vi "Audio Playback.vi"() -> ()   [LabVIEW 2020]
uses:
  support/typedefs/Playback_States.ctl
  support/typedefs/Audio CFG.ctl
  <vilib>/Dataflow_G/G-Audio/Controls/Audio File Info.ctl
  <vilib>/sound2/lvsound2.llb/Sound Output Task ID.ctl
  <vilib>/sound2/lvsound2.llb/Sampling Mode.ctl
  <vilib>/sound2/lvsound2.llb/Sound Data Format.ctl
  <vilib>/Dataflow_G/G-Audio/G-Audio.lvlib
panel:
  in  "Stop":bool
  out "#Samples":u64 format="#Samples: %d"
  in  "Audio Timeline":dbl(slide)=1.0 max=100.0 scale=0.0..100.0 scale format="%#_g %%"
  out "Playing":string="00:00:00.000"
  out "Duration":string="00:00:00.000"
  out "Bit Depth":u32 format="Bit Depth: %d"
  out "CHs":u32 format="#CH: %d"
  out "Sample Rate (Hz)":u32 format="Rate (Hz): %.0f"
  out "Audio":waveform(i16)[](graph)
  in  "Refresh List":bool
  in  "Plot Selection":T1(array[cluster])
  in  "Audio Settings":T2={"Speaker Output Device"=0, "Channels"=1, "Audio Depth"=1, "Sampling Frequncy Hz"=44100.0} {"Sampling Frequncy Hz" items=["11025"=11025.0, "22050"=22050.0, "44100"=44100.0]; "Audio Depth" items=["8", "16"]; "Channels" items=["1", "2"]; "Speaker Output Device" items=["D1918H (High Definition Audio Device)", "Speakers (2- High Definition Audio Device)"]}
  in  "Play/Pause":bool
  in  "Audio File Path":path
  in  "Modifiers":T3
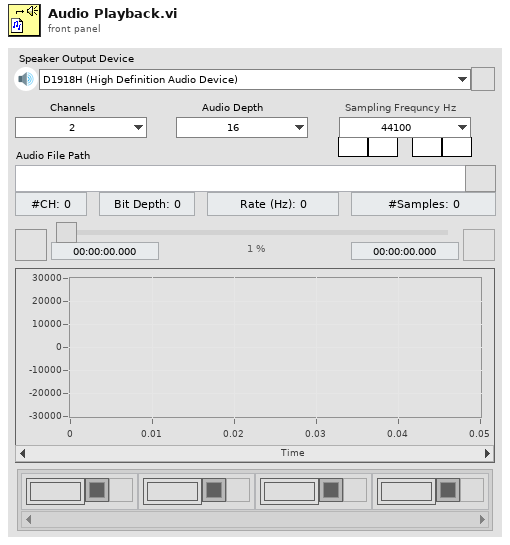
[diagram p1: front panel]
types:
  T1 = cluster{"Plot Name":string, "Plot Color":u32, "Visibility":bool}[]
  T2 = cluster{"Speaker Output Device":u32, "Channels":i32, "Audio Depth":i32, "Sampling Frequncy Hz":dbl}
  T3 = cluster{"1/4":bool, "1/2":bool, "2":bool, "4":bool}
  T4 = typedef "Audio CFG.ctl" = cluster{"CFG":cluster{"Speaker Output Device":u32, "Channels":i32, "Audio Depth":i32, "Sampling Frequncy Hz":dbl}, "Sample Length":u64, "File Info":T5, "File Refnum":refnum<file>, "File Path":path, "Task ID":T6, "Device Ready ?":bool, "Device Details":cluster{"channels":i32[], "depths":i32[], "minFreq":dbl, "maxFreq":dbl}[]}
  T5 = typedef "G-Audio.lvlib/Audio File Info.ctl" = cluster{"Sample Rate (Hz)":u32, "Channels":u32, "Bit Depth":u32}
  T6 = typedef "Sound Output Task ID.ctl" = u32
  T7 = enum8{"Enabled", "Disabled", "Disabled and Grayed Out"}
  T8 = typedef "Playback_States.ctl" = enum16{"Initialize", "Load Device List", "Load Device Info", "Respond UI", "Load File Info", "Update File Info", "Configure Speaker", "Play Audio", "Pause Audio", "Stop Audio", "Audio Finished", "Reset UI", "Handle Error", "Disable UI", "Update Plot Properties", "Select Plots", "Exit"}
  T9 = cluster{"channels":i32[], "depths":i32[], "minFreq":dbl, "maxFreq":dbl}
  T10 = cluster{"channels":i32[], "depths":i32[], "minFreq":dbl, "maxFreq":dbl}[]
  T11 = typedef "Sound Data Format.ctl" = cluster{"sample rate (S/s)":dbl, "number of channels":i32, "bits per sample":i32}
  T12 = typedef "Sampling Mode.ctl" = i32
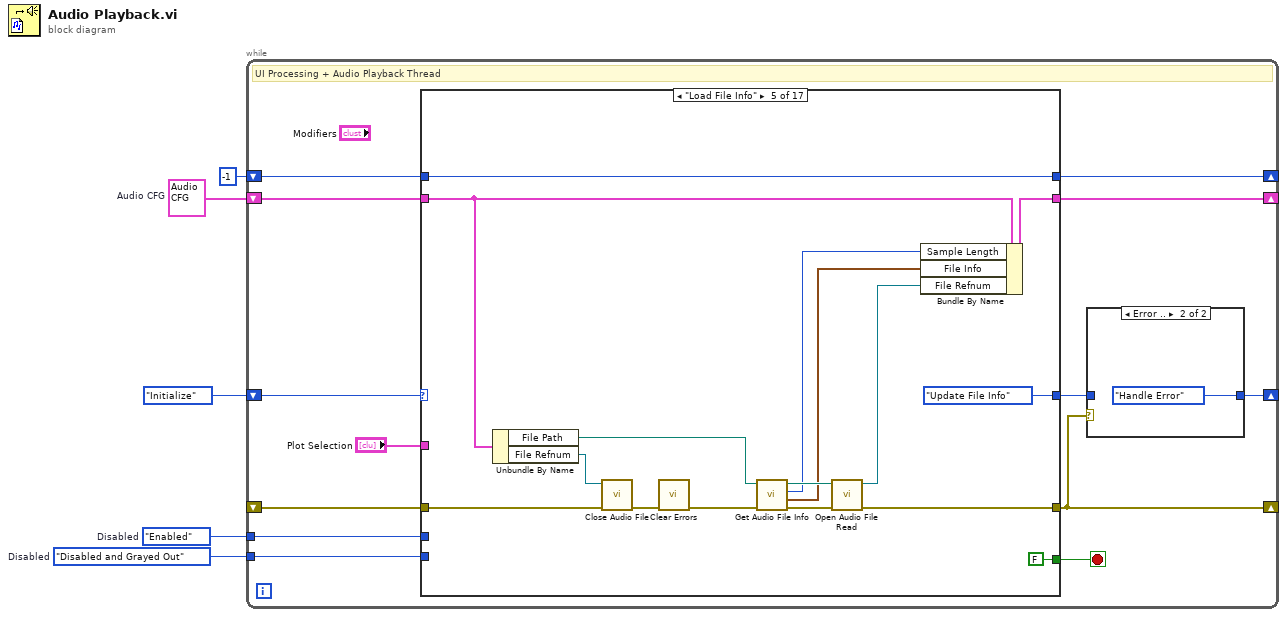
[diagram p0: block diagram]
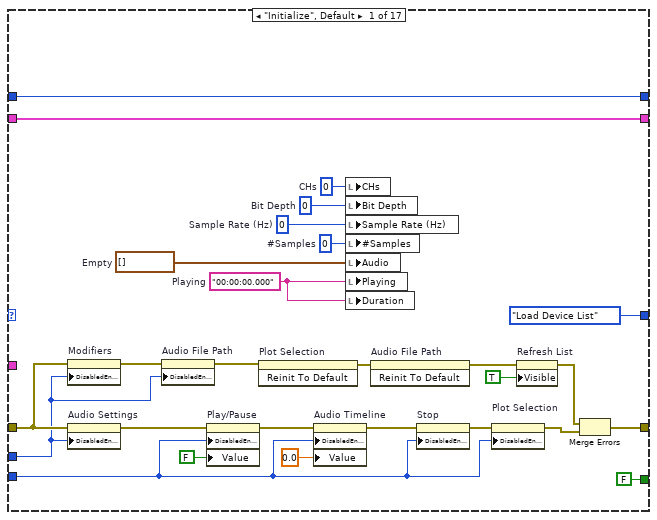
[diagram p3: hidden frame]
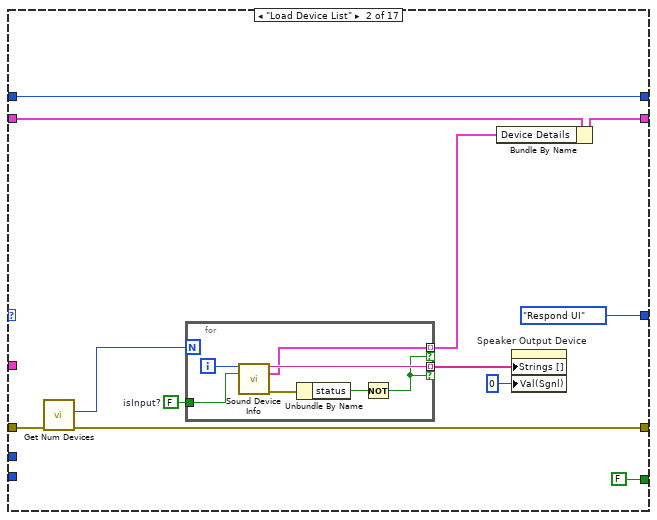
[diagram p4: hidden frame]
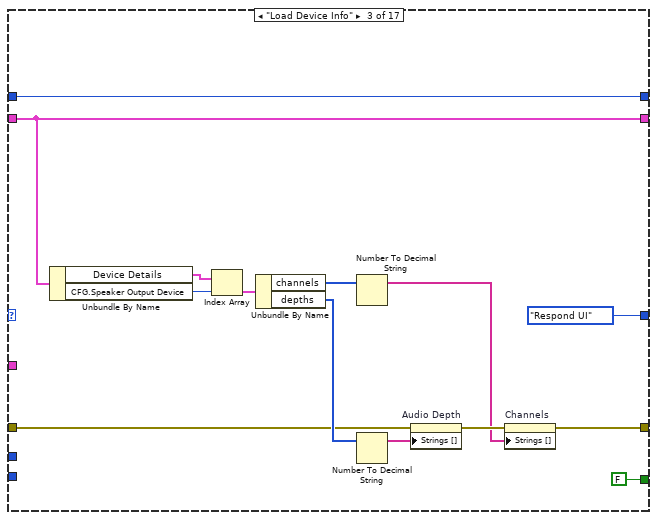
[diagram p5: hidden frame]
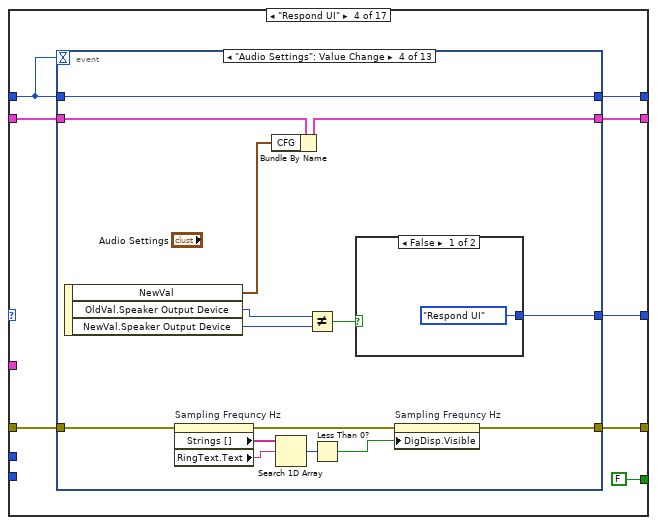
[diagram p6: hidden frame]
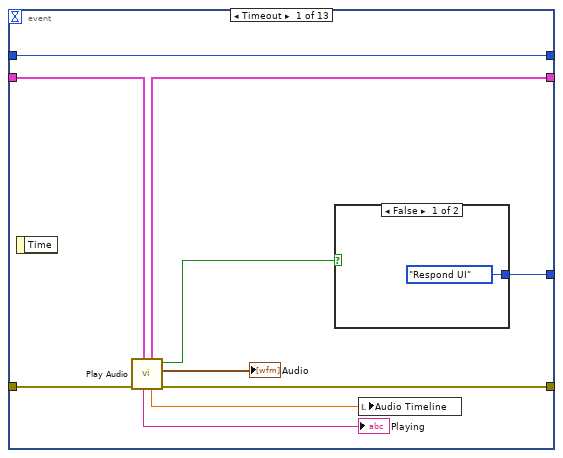
[diagram p7: hidden frame]
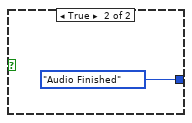
[diagram p8: hidden frame]
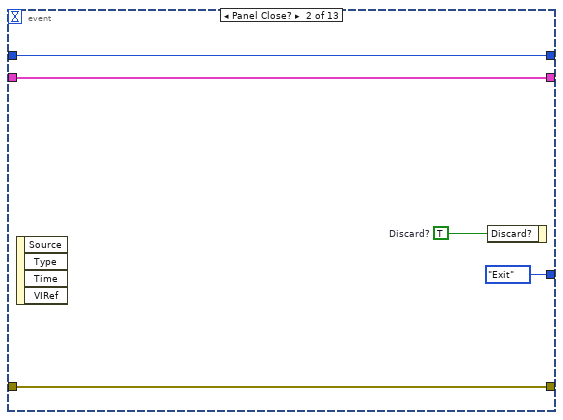
[diagram p9: hidden frame]
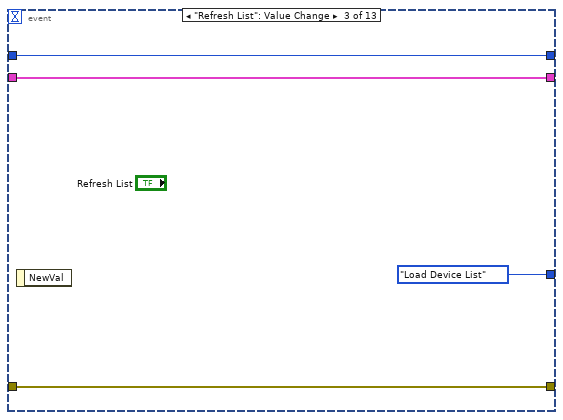
[diagram p10: hidden frame]
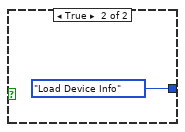
[diagram p11: hidden frame]
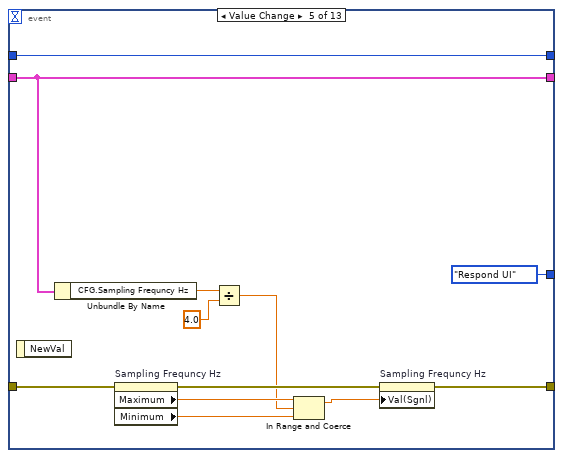
[diagram p12: hidden frame]
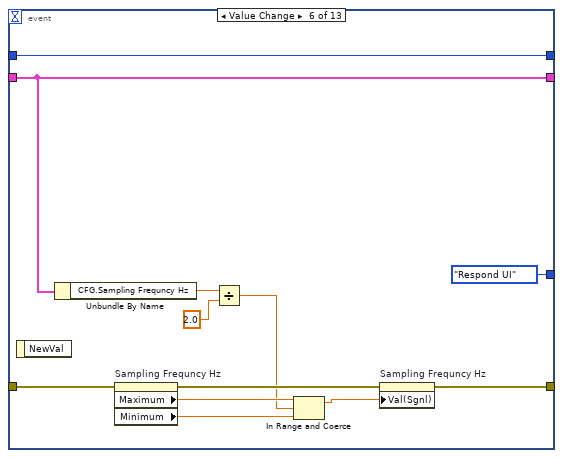
[diagram p13: hidden frame]
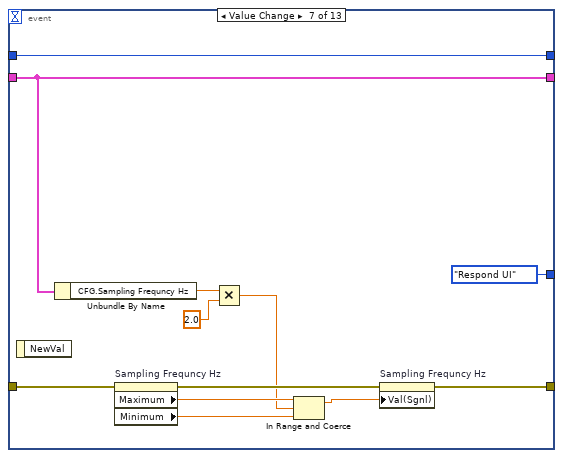
[diagram p14: hidden frame]
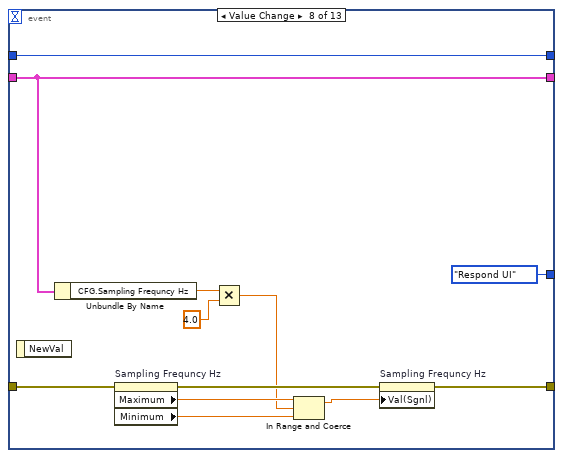
[diagram p15: hidden frame]
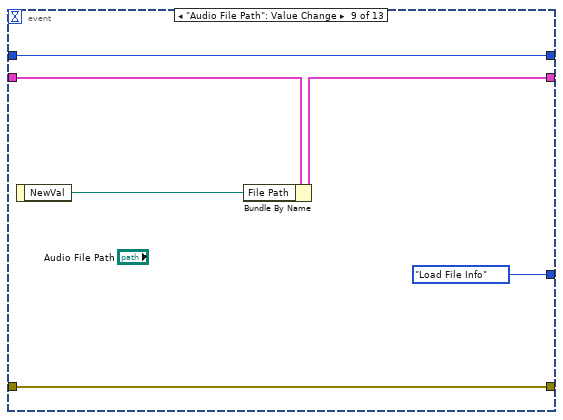
[diagram p16: hidden frame]
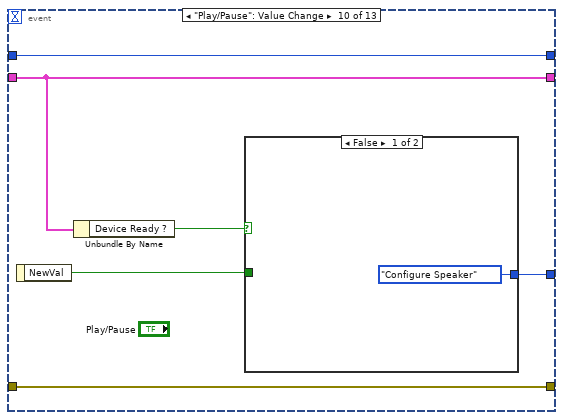
[diagram p17: hidden frame]
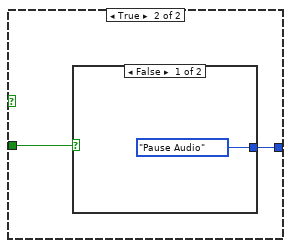
[diagram p18: hidden frame]
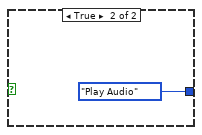
[diagram p19: hidden frame]
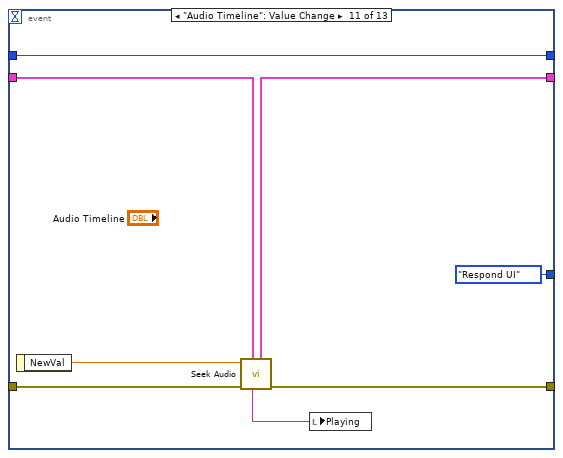
[diagram p20: hidden frame]
diagram:
  w2 = T4 {"CFG"={"Speaker Output Device"=0, "Channels"=1, "Audio Depth"=1, "Sampling Frequncy Hz"=44100.0}, "Sample Length"=0, "File Info"={"Sample Rate (Hz)"=0, "Channels"=0, "Bit Depth"=0}, "File Refnum"=refnum, "File Path"=path "", "Task ID"=0, "Device Ready ?"=FALSE, "Device Details"=[]}  # Audio CFG
  w4 = T7."Enabled"  # Disabled
  w3 = T7."Disabled and Grayed Out"  # Disabled
  n1 = while {
    shift-right: [w6] -> _
    shift-left: Playback_States."Initialize" -> [w18]
    shift-right: [w7] -> _
    shift-left: _ -> [w16]
    tunnel: w4 -> [w15]
    tunnel: w3 -> [w14]
    shift-right: [w12] -> _
    shift-left: w2 -> [w11]
    shift-right: [w9] -> _
    shift-left: -1 -> [w10]
    stop <- w17 stop-if-true
    # "UI Processing + Audio Playback Thread"
    n2 = case shown="\"Load File Info\"" w18 {
      tunnel: [FALSE FALSE FALSE FALSE FALSE FALSE FALSE FALSE FALSE FALSE FALSE FALSE FALSE FALSE FALSE FALSE TRUE] -> w17
      tunnel: [Playback_States."Load Device List" Playback_States."Respond UI" Playback_States."Respond UI" w86 Playback_States."Update File Info" Playback_States."Update Plot Properties" Playback_States."Play Audio" Playback_States."Select Plots" Playback_States."Respond UI" Playback_States."Audio Finished" Playback_States."Reset UI" Playback_States."Respond UI" Playback_States."Disable UI" Playback_States."Respond UI" Playback_States."Select Plots" Playback_States."Respond UI" Playback_States."Exit"] -> w8
      tunnel: [w45 w55 w70 w85 w219 w235 w268 w287 w295 w299 w313 w328 w344 w385 w391 w401 w421] -> w7
      tunnel: w16 -> [w24 w56 w70 w84 w232 w242 w263 w290 w295 w300 w311 w327 w343 w365 w393 w402 w425]
      tunnel: w15 -> [w21 _ _ _ _ w239 _ w280 _ _ _ w324 _ w366 _ _ _]
      tunnel: w14 -> [w33 _ _ _ _ w238 _ w272 _ _ _ w334 _ w373 _ _ _]
      tunnel: "Plot Selection" -> [_ _ _ _ _ _ _ _ _ _ _ _ _ _ _ w400 _]
      tunnel: [w42 w49 w68 w82 w229 w243 w256 w283 w294 w297 w312 w329 w345 w382 w389 w399 w419] -> w12
      tunnel: w11 -> [w42 w51 w68 w83 w224 w243 w265 w283 w294 w298 w314 w329 w346 w382 w389 w399 w419]
      tunnel: w10 -> [w41 w50 w69 w80 w225 w241 w271 _ _ w296 _ w323 w349 w381 w390 w398 w420]
      tunnel: [w41 w50 w69 w81 w225 w241 w271 0 -1 w296 -1 w323 w349 w381 w390 w398 w420] -> w9
      frame "Initialize", Default {
        w25 = "00:00:00.000"  # Playing
        w28 = u32 0  # CHs
        w29 = u32 0  # Bit Depth
        w30 = u32 0  # Sample Rate (Hz)
        w31 = u64 0  # #Samples
        w36 = waveform(i16)[] []  # Empty
        n3 = property on="Modifiers" class="Clust"(error in=w24, "DisabledEnum"=w21) -> (error out=w23:errorcluster)  [unwired: 1 in, 1 out]
        n4 = property on="Audio Settings" class="Clust (strict)"(error in=w24, "DisabledEnum"=w21) -> (error out=w40:errorcluster)  [unwired: 1 in, 1 out]
        n5 = property on="Audio File Path" class="Path"(error in=w23, "DisabledEnum"=w21) -> (error out=w22:errorcluster)  [unwired: 1 in, 1 out]
        n6 = property on="Play/Pause" class="Bool (strict)"(error in=w40, "DisabledEnum"=w33, "Value"=FALSE) -> (error out=w35:errorcluster)  [unwired: 1 in, 1 out]
        n7 = invoke on="Plot Selection" class="Arr (strict)" method="Reinit To Default"(error in=w22) -> (error out=w32:errorcluster)  [unwired: 2 in, 2 out]
        n8 = property on="Audio Timeline" class="Slide (strict)"(error in=w35, "DisabledEnum"=w33, "Value"=0.0) -> (error out=w34:errorcluster)  [unwired: 1 in, 1 out]
        n9 = local write "CHs"(w28) -> ()
        n10 = local write "Bit Depth"(w29) -> ()
        n11 = local write "Sample Rate (Hz)"(w30) -> ()
        n12 = local write "#Samples"(w31) -> ()
        n13 = local write "Audio"(w36) -> ()
        n14 = local write "Playing"(w25) -> ()
        n15 = local write "Duration"(w25) -> ()
        n16 = invoke on="Audio File Path" class="Path" method="Reinit To Default"(error in=w32) -> (error out=w26:errorcluster)  [unwired: 2 in, 2 out]
        n17 = property on="Stop" class="Bool"(error in=w34, "DisabledEnum"=w33) -> (error out=w38:errorcluster)  [unwired: 1 in, 1 out]
        n18 = property on="Plot Selection" class="Arr (strict)"(error in=w38, "DisabledEnum"=w33) -> (error out=w39:errorcluster)  [unwired: 1 in, 1 out]
        n19 = property on="Refresh List" class="Bool"(error in=w26, "Visible"=TRUE) -> (error out=w44:errorcluster)  [unwired: 1 in, 1 out]
        n20 = Merge Errors(w44, w39) -> (w45:errorcluster)
      }
      frame "Load Device List" {
        w53 = FALSE  # isInput?
        n21 = call <vilib>:"Get Num Devices.vi"("error in (no error)"=w56) -> ("error out"=w55:errorcluster, "Number of Output Devices"=w54:i32)  [unwired: 8 in, 1 out]
        n22 = for {
          N: w54 -> [_]
          tunnel: [w65] -> w57 mode=indexing if=w61
          tunnel: [w64] -> w48 mode=indexing if=w61
          tunnel: w53 -> [w60]
          i -> [w66]
          n23 = call <vilib>:"Sound Device Info.vi"("device"=w66, "isInput?"=w60) -> ("Device Name"=w65:string, "Capabilities"=w64:T9, "error out"=w63:errorcluster)  [unwired: 11 in]
          n24 = Unbundle By Name(w63) -> ("status"=w62:bool)
          n25 = Not(x=w62) -> (.not. x?=w61:bool)
        }
        n26 = Bundle By Name(cluster=w51, "Device Details"=w48) -> (w49:T4)
        n27 = property on="Speaker Output Device" class="Ring (strict)"("Strings []"=w57, "Val(Sgnl)"=u32 0) -> ()  [unwired: 2 in, 2 out]
      }
      frame "Load Device Info" {
        n28 = Unbundle By Name(w68) -> ("Device Details"=w67:T10, "CFG.Speaker Output Device"=w76:u32)
        n29 = Index Array(array=w67, index=w76) -> (element=w75:T9)
        n30 = Unbundle By Name(w75) -> ("channels"=w73:i32[], "depths"=w74:i32[])
        n31 = Number To Decimal String(number=w73) -> (decimal integer string=w72:string[])  [unwired: 1 in]
        n32 = Number To Decimal String(number=w74) -> (decimal integer string=w71:string[])  [unwired: 1 in]
        n33 = property on="Audio Depth" class="Ring (strict)"("Strings []"=w71) -> (error out=w77:errorcluster)  [unwired: 2 in, 1 out]
        n34 = property on="Channels" class="Ring (strict)"(error in=w77, "Strings []"=w72) -> ()  [unwired: 1 in, 2 out]
      }
      frame "Respond UI" {
        n35 = event shown="[3] \"Audio Settings\": Value Change" {
          selector: _ -> [_ _ _ _ _ _ _ _ _ _ _ _ _]
          dyn-events: _ -> [_ _ _ _ _ _ _ _ _ _ _ _ _]
          timeout: w80 -> [_ _ _ _ _ _ _ _ _ _ _ _ _]
          tunnel: [w97 Playback_States."Exit" Playback_States."Load Device List" w122 Playback_States."Respond UI" Playback_States."Respond UI" Playback_States."Respond UI" Playback_States."Respond UI" Playback_States."Load File Info" w183 Playback_States."Respond UI" Playback_States."Stop Audio" w210] -> w86
          tunnel: [w94 w100 w108 w110 w132 w144 w156 w168 w177 w185 w195 w202 w208] -> w85
          tunnel: w84 -> [w95 w100 w108 w115 w131 w143 w155 w167 w177 w185 w198 w202 w209]
          tunnel: w83 -> [w93 w104 w107 w116 w133 w145 w157 w169 w179 w181 w194 w201 w212]
          tunnel: [w92 w104 w107 w121 w133 w145 w157 w169 w175 w181 w193 w201 w212] -> w82
          tunnel: [w96 w103 w106 w123 w137 w149 w161 w173 w178 w184 w197 w200 w211] -> w81
          tunnel: w80 -> [w96 w103 w106 w123 w137 w149 w161 w173 w178 w184 w197 w200 w211]
          event Timeout {
            n36 = event-data() -> ()  [unwired: 1 in, 1 out]
            n37 = call "Play Audio.vi"("Audio CFG in"=w93, "error in (no error)"=w95) -> ("error out"=w94:errorcluster, "Now Playing"=→"Audio":waveform(i16)[], "Completed ?"=w91:bool, "Now Playing (%)"=w89:dbl, "Audio CFG out"=w92:T4, "Now Playing (Time)"=→"Playing":string)  [unwired: 4 in]
            n38 = case shown="False" w91 {
              tunnel: [Playback_States."Respond UI" Playback_States."Audio Finished"] -> w97
              frame False {
              }
              frame True {
              }
            }
            n39 = local write "Audio Timeline"(w89) -> ()
          }
          event Panel Close? {
            w101 = TRUE  # Discard?
            n40 = event-data() -> ()  [unwired: 1 in, 4 out]
            n41 = event-data("Discard?"=w101) -> ()  [unwired: 1 in, 1 out]
          }
          event "Refresh List": Value Change {
            n42 = event-data() -> ()  [unwired: 1 in, 1 out]
          }
          event "Audio Settings": Value Change {
            n43 = event-data() -> ("NewVal"=w120:T2, "OldVal.Speaker Output Device"=w119:u32, "NewVal.Speaker Output Device"=w118:u32)  [unwired: 1 in]
            n44 = property on="Sampling Frequncy Hz" class="Ring (strict)"(error in=w115) -> (error out=w111:errorcluster, "Strings []"=w113:string[], "RingText.Text"=w114:string)  [unwired: 1 in, 1 out]
            n45 = Bundle By Name(cluster=w116, "CFG"=w120) -> (w121:T4)
            n46 = Search 1D Array(1D array=w113, element=w114) -> (index of element=w112:i32)  [unwired: 1 in]
            n47 = Not Equal?(x=w119, y=w118) -> (x != y?=w117:bool)
            n48 = Less Than 0?(x=w112) -> (x < 0?=w109:bool)
            n49 = case shown="False" w117 {
              tunnel: [Playback_States."Respond UI" Playback_States."Load Device Info"] -> w122
              frame False {
              }
              frame True {
              }
            }
            n50 = property on="Sampling Frequncy Hz" class="Ring (strict)"(error in=w111, "DigDisp.Visible"=w109) -> (error out=w110:errorcluster)  [unwired: 1 in, 1 out]
          }
          event "Modifiers.1/4": Value Change {
            n51 = event-data() -> ()  [unwired: 1 in, 1 out]
            n52 = Unbundle By Name(w133) -> ("CFG.Sampling Frequncy Hz"=w135:dbl)
            n53 = property on="Sampling Frequncy Hz" class="Ring (strict)"(error in=w131) -> (error out=w130:errorcluster, "Maximum"=w129:dbl, "Minimum"=w128:dbl)  [unwired: 1 in, 1 out]
            n54 = Divide(x=w135, y=4.0) -> (x/y=w127:dbl)
            n55 = In Range and Coerce(upper limit=w129, x=w127, lower limit=w128) -> (coerced(x)=w126:dbl)  [unwired: 1 out]
            n56 = property on="Sampling Frequncy Hz" class="Ring (strict)"(error in=w130, "Val(Sgnl)"=w126) -> (error out=w132:errorcluster)  [unwired: 1 in, 1 out]
          }
          event "Modifiers.1/2": Value Change {
            n57 = event-data() -> ()  [unwired: 1 in, 1 out]
            n58 = Unbundle By Name(w145) -> ("CFG.Sampling Frequncy Hz"=w147:dbl)
            n59 = property on="Sampling Frequncy Hz" class="Ring (strict)"(error in=w143) -> (error out=w142:errorcluster, "Maximum"=w141:dbl, "Minimum"=w140:dbl)  [unwired: 1 in, 1 out]
            n60 = Divide(x=w147, y=2.0) -> (x/y=w139:dbl)
            n61 = In Range and Coerce(upper limit=w141, x=w139, lower limit=w140) -> (coerced(x)=w138:dbl)  [unwired: 1 out]
            n62 = property on="Sampling Frequncy Hz" class="Ring (strict)"(error in=w142, "Val(Sgnl)"=w138) -> (error out=w144:errorcluster)  [unwired: 1 in, 1 out]
          }
          event "Modifiers.2": Value Change {
            n63 = event-data() -> ()  [unwired: 1 in, 1 out]
            n64 = Unbundle By Name(w157) -> ("CFG.Sampling Frequncy Hz"=w159:dbl)
            n65 = property on="Sampling Frequncy Hz" class="Ring (strict)"(error in=w155) -> (error out=w154:errorcluster, "Maximum"=w153:dbl, "Minimum"=w152:dbl)  [unwired: 1 in, 1 out]
            n66 = Multiply(x=w159, y=2.0) -> (x*y=w151:dbl)
            n67 = In Range and Coerce(upper limit=w153, x=w151, lower limit=w152) -> (coerced(x)=w150:dbl)  [unwired: 1 out]
            n68 = property on="Sampling Frequncy Hz" class="Ring (strict)"(error in=w154, "Val(Sgnl)"=w150) -> (error out=w156:errorcluster)  [unwired: 1 in, 1 out]
          }
          event "Modifiers.4": Value Change {
            n69 = event-data() -> ()  [unwired: 1 in, 1 out]
            n70 = Unbundle By Name(w169) -> ("CFG.Sampling Frequncy Hz"=w171:dbl)
            n71 = property on="Sampling Frequncy Hz" class="Ring (strict)"(error in=w167) -> (error out=w166:errorcluster, "Maximum"=w165:dbl, "Minimum"=w164:dbl)  [unwired: 1 in, 1 out]
            n72 = Multiply(x=w171, y=4.0) -> (x*y=w163:dbl)
            n73 = In Range and Coerce(upper limit=w165, x=w163, lower limit=w164) -> (coerced(x)=w162:dbl)  [unwired: 1 out]
            n74 = property on="Sampling Frequncy Hz" class="Ring (strict)"(error in=w166, "Val(Sgnl)"=w162) -> (error out=w168:errorcluster)  [unwired: 1 in, 1 out]
          }
          event "Audio File Path": Value Change {
            n75 = event-data() -> ("NewVal"=w174:path)  [unwired: 1 in]
            n76 = Bundle By Name(cluster=w179, "File Path"=w174) -> (w175:T4)
          }
          event "Play/Pause": Value Change {
            n77 = event-data() -> ("NewVal"=w182:bool)  [unwired: 1 in]
            n78 = Unbundle By Name(w181) -> ("Device Ready ?"=w180:bool)
            n79 = case shown="False" w180 {
              tunnel: [Playback_States."Configure Speaker" w188] -> w183
              tunnel: w182 -> [_ w187]
              frame False {
              }
              frame True {
                n80 = case shown="False" w187 {
                  tunnel: [Playback_States."Pause Audio" Playback_States."Play Audio"] -> w188
                  frame False {
                  }
                  frame True {
                  }
                }
              }
            }
          }
          event "Audio Timeline": Value Change {
            n81 = event-data() -> ("NewVal"=w192:dbl)  [unwired: 1 in]
            n82 = call "Seek Audio.vi"("Audio CFG in"=w194, "error in (no error)"=w198, "Seek Position %"=w192) -> ("error out"=w195:errorcluster, "Audio CFG out"=w193:T4, "Now Playing (Time)"=w191:string)  [unwired: 5 in, 1 out]
            n83 = local write "Playing"(w191) -> ()
          }
          event "Stop": Value Change {
            n84 = event-data() -> ()  [unwired: 1 in, 1 out]
          }
          event "Plot Selection": Value Change {
            n85 = event-data() -> ("NewVal"=w207:T1, "OldVal"=w206:T1)  [unwired: 1 in]
            n86 = Array Size(array=w207) -> (size(s)=w205:i32)
            n87 = Array Size(array=w206) -> (size(s)=w204:i32)
            n88 = Not Equal?(x=w205, y=w204) -> (x != y?=w203:bool)
            n89 = case shown="False" w203 {
              tunnel: [Playback_States."Select Plots" Playback_States."Respond UI"] -> w210
              tunnel: w209 -> [w213 w217]
              tunnel: [w213 w216] -> w208
              tunnel: w206 -> [_ w215]
              frame False {
              }
              frame True {
                n90 = property on="Plot Selection" class="Arr (strict)"(error in=w217, "Value"=w215) -> (error out=w216:errorcluster)  [unwired: 1 in, 1 out]
              }
            }
          }
        }
      }
      frame "Load File Info" {
        n91 = Unbundle By Name(w224) -> ("File Path"=w223:path, "File Refnum"=w221:refnum<file>)
        n92 = call <vilib>:"Close Audio File.vi"("error in (no error)"=w232, "Audio File Refnum In"=w221) -> ("error out"=w222:errorcluster)  [unwired: 9 in]
        n93 = call <vilib>:"Clear Errors.vi"("error in (no error)"=w222) -> ("error out"=w220:errorcluster)  [unwired: 5 in, 1 out]
        n94 = call <vilib>:"Get Audio File Info.vi"("error in (no error)"=w220, "Path In"=w223) -> ("error out"=w231:errorcluster, "Audio File Info"=w227:T5, "Sample Length"=w228:u64, "Path Out"=w230:path)  [unwired: 6 in]
        n95 = call <vilib>:"Open Audio File Read.vi"("error in (no error)"=w231, "Path"=w230) -> ("error out"=w219:errorcluster, "Audio File Refnum"=w226:refnum<file>)  [unwired: 8 in]
        n96 = Bundle By Name(cluster=w224, "Sample Length"=w228, "File Info"=w227, "File Refnum"=w226) -> (w229:T4)
      }
      frame "Update File Info" {
        w237 = waveform(i16)[] []  # Empty
        n97 = property on="Play/Pause" class="Bool (strict)"(error in=w242, "DisabledEnum"=w239) -> (error out=w240:errorcluster)  [unwired: 1 in, 1 out]
        n98 = Unbundle By Name(w243) -> ("Sample Length"=w246:u64, "File Info.Sample Rate (Hz)"=w236:u32, "File Info.Channels"=→"CHs":u32, "File Info.Bit Depth"=→"Bit Depth":u32)
        "#Samples" <- w246
        "Sample Rate (Hz)" <- w236
        n99 = property on="Stop" class="Bool"(error in=w240, "DisabledEnum"=w238) -> (error out=w235:errorcluster)  [unwired: 1 in, 1 out]
        n100 = Divide(x=w246, y=w236) -> (x/y=w249:dbl)
        n101 = Format Date/Time String(time format string (%c)="%H:%M:%S%3u", seconds (now)=w249, UTC format=TRUE) -> (date/time string=→"Duration":string)
        n102 = local write "Audio"(w237) -> ()
      }
      frame "Configure Speaker" {
        w261 = T11 {"sample rate (S/s)"=22050.0, "number of channels"=2, "bits per sample"=16}  # sound format
        w266 = 2048  # number of samples/ch
        w267 = T12 1 items=["Finite Samples", "Continuous Samples"]  # sample mode
        n103 = Unbundle By Name(w265) -> ("Device Details"=w253:T10, "CFG"=w264:T2)
        n104 = call "Build_Device_Details.vi"("Audio Settings"=w264, "Audio Device Details"=w253) -> ("Sampling Frequncy Hz"=w259:dbl, "Depth"=w258:i32, "Channel"=w257:i32, "Device ID"=w262:u32)  [unwired: 4 in, 2 out]
        n105 = Bundle By Name(cluster=w261, "number of channels"=w257, "bits per sample"=w258, "sample rate (S/s)"=w259) -> (w260:T11)
        n106 = call <vilib>:"Sound Output Configure.vi"("number of samples/ch"=w266, "sample mode"=w267, "error in (no error)"=w263, "sound format"=w260, "device ID"=w262) -> ("error out"=w268:errorcluster, "task ID"=w255:T6)  [unwired: 5 in]
        n107 = Bundle By Name(cluster=w265, "Task ID"=w255, "Device Ready ?"=TRUE) -> (w256:T4)
      }
      frame "Play Audio" {
        n108 = call <vilib>:"Set Busy.vi"("error in (no error)"=w290) -> ("error out"=w276:errorcluster)  [unwired: 9 in, 1 out]
        n109 = property on="Play/Pause" class="Bool (strict)"(error in=w276, "DisabledEnum"=w280) -> (error out=w284:errorcluster)  [unwired: 1 in, 1 out]
        n110 = property on="Audio Timeline" class="Slide (strict)"(error in=w276, "DisabledEnum"=w280) -> (error out=w281:errorcluster)  [unwired: 1 in, 1 out]
        n111 = property on="Plot Selection" class="Arr (strict)"(error in=w284, "DisabledEnum"=w280) -> (error out=w274:errorcluster)  [unwired: 1 in, 1 out]
        n112 = property on="Stop" class="Bool"(error in=w281, "DisabledEnum"=w280) -> (error out=w275:errorcluster)  [unwired: 1 in, 1 out]
        n113 = property on="Audio File Path" class="Path"(error in=w274, "DisabledEnum"=w272) -> (error out=w273:errorcluster)  [unwired: 1 in, 1 out]
        n114 = property on="Refresh List" class="Bool"(error in=w275, "Visible"=FALSE) -> (error out=w279:errorcluster)  [unwired: 1 in, 1 out]
        n115 = property on="Audio Settings" class="Clust (strict)"(error in=w279, "DisabledEnum"=w272) -> (error out=w278:errorcluster)  [unwired: 1 in, 1 out]
        n116 = property on="Modifiers" class="Clust"(error in=w273, "DisabledEnum"=w272) -> (error out=w277:errorcluster)  [unwired: 1 in, 1 out]
        n117 = Merge Errors(w278, w277) -> (w285:errorcluster)
        n118 = call <vilib>:"Unset Busy.vi"("error in (no error)"=w285) -> ("error out"=w287:errorcluster)  [unwired: 10 in]
      }
      frame "Pause Audio" {
      }
      frame "Stop Audio" {
        n119 = in-place {
          in-place-border: w300 -> [w308]
          in-place-border: [w303] -> w299
          n120 = in-place-cluster #1(w298) -> ("Task ID"=w306:T6)  [unwired: 1 out]
          n121 = call <vilib>:"Sound Output Wait.vi"("error in (no error)"=w308, "task ID"=w306) -> ("error out"=w310:errorcluster, "task ID out"=w309:T6)  [unwired: 8 in]
          n122 = call <vilib>:"Sound Output Clear.vi"("error in (no error)"=w310, "task ID"=w309) -> ("error out"=w304:errorcluster)  [unwired: 9 in]
          n123 = call <vilib>:"Clear Errors.vi"("error in (no error)"=w304) -> ("error out"=w303:errorcluster)  [unwired: 5 in, 1 out]
          n124 = in-place-cluster #1("Device Ready ?"=FALSE, "Task ID"=T6 0) -> (w297:T4)
        }
      }
      frame "Audio Finished" {
        n125 = in-place {
          in-place-border: w311 -> [w318]
          in-place-border: [w322] -> w313
          w321 = u64 0  # Seek Position
          n126 = in-place-cluster #2(w314) -> ("File Refnum"=w320:refnum<file>)
          n127 = call <vilib>:"Seek Audio File.vi"("error in (no error)"=w318, "Seek Position"=w321, "Audio File Refnum In"=w320) -> ("error out"=w322:errorcluster, "Audio File Refnum Out"=w319:refnum<file>)  [unwired: 7 in]
          n128 = in-place-cluster #2("File Refnum"=w319) -> (w312:T4)
        }
      }
      frame "Reset UI" {
        w332 = "00:00:00.000"  # Playing
        w337 = waveform(i16)[] []  # Empty
        n129 = property on="Modifiers" class="Clust"(error in=w327, "DisabledEnum"=w324) -> (error out=w326:errorcluster)  [unwired: 1 in, 1 out]
        n130 = property on="Audio Settings" class="Clust (strict)"(error in=w327, "DisabledEnum"=w324) -> (error out=w339:errorcluster)  [unwired: 1 in, 1 out]
        n131 = property on="Audio File Path" class="Path"(error in=w326, "DisabledEnum"=w324) -> (error out=w325:errorcluster)  [unwired: 1 in, 1 out]
        n132 = property on="Play/Pause" class="Bool (strict)"(error in=w339, "DisabledEnum"=w324, "Value"=FALSE) -> (error out=w336:errorcluster)  [unwired: 1 in, 1 out]
        n133 = property on="Audio Timeline" class="Slide (strict)"(error in=w336, "DisabledEnum"=w334, "Value"=0.0) -> (error out=w335:errorcluster)  [unwired: 1 in, 1 out]
        n134 = local write "Audio"(w337) -> ()
        n135 = local write "Playing"(w332) -> ()
        n136 = property on="Stop" class="Bool"(error in=w335, "DisabledEnum"=w334) -> (error out=w331:errorcluster)  [unwired: 1 in, 1 out]
        n137 = property on="Refresh List" class="Bool"(error in=w331, "Visible"=TRUE) -> (error out=w330:errorcluster)  [unwired: 1 in, 1 out]
        n138 = Merge Errors(w325, w330) -> (w328:errorcluster)
      }
      frame "Handle Error" {
        n139 = in-place {
          in-place-border: [w350] -> w344
          in-place-border: w343 -> [w360]
          w352 = refnum<file> refnum  # File Refnum
          w356 = T6 0  # Task ID
          n140 = in-place-cluster #3(w346) -> ("File Refnum"=w353:refnum<file>, "Task ID"=w357:T6)  [unwired: 1 out]
          n141 = call <vilib>:"Simple Error Handler.vi"("error in (no error)"=w360) -> ("error out"=w359:errorcluster)  [unwired: 4 in, 4 out]
          n142 = call <vilib>:"Clear Errors.vi"("error in (no error)"=w359) -> ("error out"=w358:errorcluster)  [unwired: 5 in, 1 out]
          n143 = call <vilib>:"Sound Output Clear.vi"("error in (no error)"=w358, "task ID"=w357) -> ("error out"=w355:errorcluster)  [unwired: 9 in]
          n144 = call <vilib>:"Clear Errors.vi"("error in (no error)"=w355) -> ("error out"=w354:errorcluster)  [unwired: 5 in, 1 out]
          n145 = call <vilib>:"Close Audio File.vi"("error in (no error)"=w354, "Audio File Refnum In"=w353) -> ("error out"=w351:errorcluster)  [unwired: 9 in]
          n146 = call <vilib>:"Clear Errors.vi"("error in (no error)"=w351) -> ("error out"=w350:errorcluster)  [unwired: 5 in, 1 out]
          n147 = in-place-cluster #3("Device Ready ?"=FALSE, "File Refnum"=w352, "Task ID"=w356) -> (w345:T4)
        }
      }
      frame "Disable UI" {
        w367 = "00:00:00.000"  # Playing
        w369 = u32 0  # CHs
        w370 = u32 0  # Bit Depth
        w371 = u32 0  # Sample Rate (Hz)
        w372 = u64 0  # #Samples
        w376 = waveform(i16)[] []  # Empty
        n148 = property on="Modifiers" class="Clust"(error in=w365, "DisabledEnum"=w366) -> (error out=w364:errorcluster)  [unwired: 1 in, 1 out]
        n149 = property on="Audio Settings" class="Clust (strict)"(error in=w365, "DisabledEnum"=w366) -> (error out=w380:errorcluster)  [unwired: 1 in, 1 out]
        n150 = invoke on="Plot Selection" class="Arr (strict)" method="Reinit To Default"(error in=w364) -> (error out=w363:errorcluster)  [unwired: 2 in, 2 out]
        n151 = property on="Play/Pause" class="Bool (strict)"(error in=w380, "DisabledEnum"=w373, "Value"=FALSE) -> (error out=w375:errorcluster)  [unwired: 1 in, 1 out]
        n152 = invoke on="Audio File Path" class="Path" method="Reinit To Default"(error in=w363) -> (error out=w362:errorcluster)  [unwired: 2 in, 2 out]
        n153 = property on="Audio Timeline" class="Slide (strict)"(error in=w375, "DisabledEnum"=w373, "Value"=0.0) -> (error out=w374:errorcluster)  [unwired: 1 in, 1 out]
        n154 = local write "CHs"(w369) -> ()
        n155 = local write "Bit Depth"(w370) -> ()
        n156 = local write "Sample Rate (Hz)"(w371) -> ()
        n157 = local write "#Samples"(w372) -> ()
        n158 = local write "Audio"(w376) -> ()
        n159 = local write "Playing"(w367) -> ()
        n160 = local write "Duration"(w367) -> ()
        n161 = property on="Stop" class="Bool"(error in=w374, "DisabledEnum"=w373) -> (error out=w378:errorcluster)  [unwired: 1 in, 1 out]
        n162 = property on="Refresh List" class="Bool"(error in=w362, "Visible"=TRUE) -> (error out=w384:errorcluster)  [unwired: 1 in, 1 out]
        n163 = property on="Plot Selection" class="Arr (strict)"(error in=w378, "DisabledEnum"=w373) -> (error out=w379:errorcluster)  [unwired: 1 in, 1 out]
        n164 = Merge Errors(w384, w379) -> (w385:errorcluster)
      }
      frame "Update Plot Properties" {
        n165 = Unbundle By Name(w389) -> ("File Info"=w388:T5)
        n166 = call <vilib>:"Set Busy.vi"("error in (no error)"=w393) -> ("error out"=w392:errorcluster)  [unwired: 9 in, 1 out]
        n167 = call "Build_Plot_Selection-Playback.vi"("File Info"=w388, "error in (no error)"=w392) -> ("error out"=w394:errorcluster, "Plot Selection"=w395:T1)  [unwired: 8 in]
        n168 = local write "Plot Selection"(w395) -> ()
        n169 = call <vilib>:"Unset Busy.vi"("error in (no error)"=w394) -> ("error out"=w391:errorcluster)  [unwired: 10 in]
      }
      frame "Select Plots" {
        n170 = for {
          shift-right: [w412] -> w401
          shift-left: w402 -> [w406]
          tunnel: w400 -> [w411] mode=indexing
          i -> [w405]
          n171 = Unbundle By Name(w411) -> ("Plot Name"=w410:string, "Plot Color"=w409:u32, "Visibility"=w408:bool)
          n172 = property on="Audio" class="WFGraph (strict)"(error in=w406, "Active Plot"=w405) -> (error out=w407:errorcluster)  [unwired: 1 in, 1 out]
          n173 = property on="Audio" class="WFGraph (strict)"(error in=w407, "Plot.Plot Name"=w410, "Plot.Plot Color"=w409, "Plot.Visible?"=w408) -> (error out=w412:errorcluster)  [unwired: 1 in, 1 out]
        }
      }
      frame "Exit" {
        n174 = call <vilib>:"Set Busy.vi"("error in (no error)"=w425) -> ("error out"=w422:errorcluster)  [unwired: 9 in, 1 out]
        n175 = Unbundle By Name(w419) -> ("Device Ready ?"=w413:bool, "Task ID"=w415:T6, "File Refnum"=w417:refnum<file>)
        n176 = call <vilib>:"Close Audio File.vi"("error in (no error)"=w422, "Audio File Refnum In"=w417) -> ("error out"=w418:errorcluster)  [unwired: 9 in]
        n177 = call <vilib>:"Clear Errors.vi"("error in (no error)"=w418) -> ("error out"=w416:errorcluster)  [unwired: 5 in, 1 out]
        n178 = case shown="False" w413 {
          tunnel: w416 -> [w426 w431]
          tunnel: w415 -> [_ w430]
          tunnel: [w426 w428] -> w414
          frame False {
          }
          frame True {
            n179 = call <vilib>:"Sound Output Wait.vi"("error in (no error)"=w431, "task ID"=w430) -> ("error out"=w429:errorcluster, "task ID out"=w427:T6)  [unwired: 8 in]
            n180 = call <vilib>:"Sound Output Clear.vi"("error in (no error)"=w429, "task ID"=w427) -> ("error out"=w428:errorcluster)  [unwired: 9 in]
          }
        }
        n181 = call <vilib>:"Unset Busy.vi"("error in (no error)"=w414) -> ("error out"=w421:errorcluster)  [unwired: 10 in]
      }
    }
    n182 = case shown="Error .." w7 {
      tunnel: w8 -> [w19 _]
      tunnel: [w19 Playback_States."Handle Error"] -> w6
      frame No Error {
      }
      frame Error {
      }
    }
  }
